vi "read ad x.vi"(8 "error in (no error)":errorcluster, 11 "x":u16) -> (0 "error out":errorcluster, 3 "function return":u16)   [LabVIEW 2015, in "SCANalone4x64.lvlib"]
doc: "__declspec(dllimport) unsigned short __stdcall read_ad_x(unsigned short x);"
uses:
  <userlib>/SCANalone4x64/SCANalone4x64.lvlib
  <userlib>/SCANalone4x64/SCANalone4x64.dll
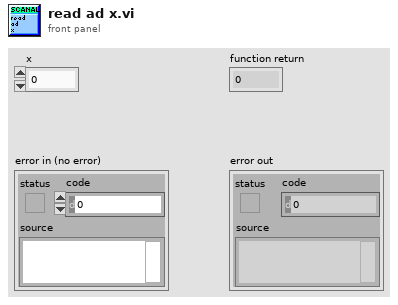
[diagram p1: front panel]
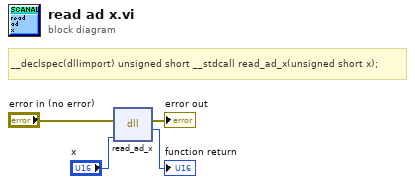
[diagram p0: block diagram]
diagram:
  # "__declspec(dllimport) unsigned short __stdcall read_ad_x(unsigned short x);"
  n1 = dll-call lib="C:/Program Files/National Instruments/LabVIEW 2015/user.lib/SCANalone4x64/SCANalone4x64.*" fn="read_ad_x"(error in="error in (no error)", "x"="x") -> (error out=→"error out":errorcluster, →"function return":u16)  [unwired: 3 in, 1 out]
